vi "9239_1 - test.vi"() -> ()   [LabVIEW 2014]
uses:
  <vilib>/Platform/TimedLoop/XDataNode/timing_clust.ctl
  <vilib>/Platform/TimedLoop/XDataNode/nitl_modes.ctl
  <vilib>/Platform/TimedLoop/XDataNode/wakeup.ctl
  <vilib>/Platform/TimedLoop/XDataNode/XDataNode.xnode
  <vilib>/Platform/TimedLoop/XDataNode/XDNodeRunTimeDep.lvlib
panel:
  out "已采样数量":dbl
  out "a1通道零漂采集":dynamicdata(graph)
  in  "路径":path=path "test"
  out "波形图":dynamicdata(graph)
  out "时间":string
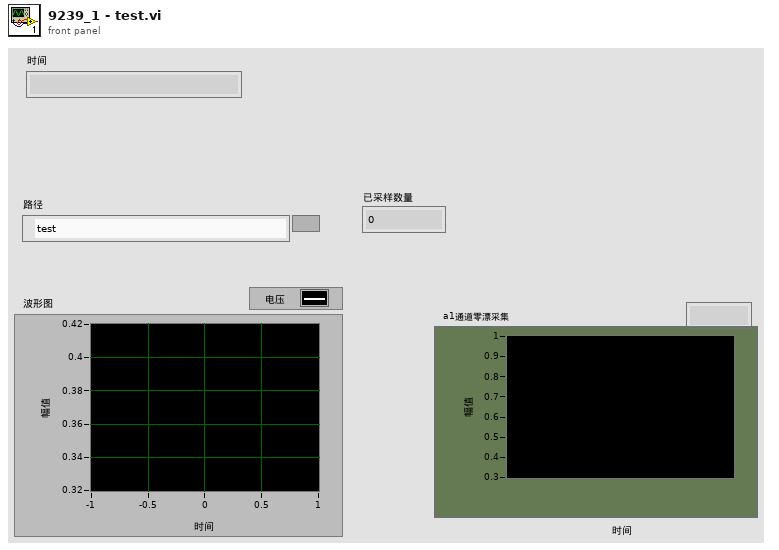
[diagram p1: front panel]
types:
  T1 = enum16{"open", "open or create", "create or replace", "create", "open (read-only)"}
  T2 = typedef "XDNodeRunTimeDep.lvlib/timing_clust.ctl" = cluster{"Expected End [f-1]":u64, "Actual End [f-1]":u64, "Finished Late? [f-1]":bool, "Expected End [i-1]":u64, "Actual End [i-1]":u64, "Finished Late? [i-1]":bool, "Expected Start [i]":u64, "Actual Start [i]":u64, "Expected Start [f]":u64, "Actual Start [f]":u64, "Source Name":string, "Structure Name":string, "Period":i64, "Deadline":i64, "Offset":i64, "Start":i64, "Priority":i32, "Timeout":i32, "Mode":T3, "Wakeup Reason":T4, "Error":errorcluster, "Source Type":string, "Secondary Source Type":string, "Global End Time":u64, "Global Start Time":u64, "Frame Duration":u64, "Iteration Duration":u64, "Assigned CPU":i32, "I/O Scan Engine Mode":u32}
  T3 = typedef "XDNodeRunTimeDep.lvlib/nitl_modes.ctl" = enum32{"No Change", "Process missed periods, maintain original phase", "Discard missed periods, maintain original phase", "Process missed periods, ignore original phase", "Discard missed periods, ignore original phase"}
  T4 = typedef "XDNodeRunTimeDep.lvlib/wakeup.ctl" = enum32{"Normal", "Aborted", "Asynchronous wakeup", "Timing source error", "Timed loop error", "Timeout"}
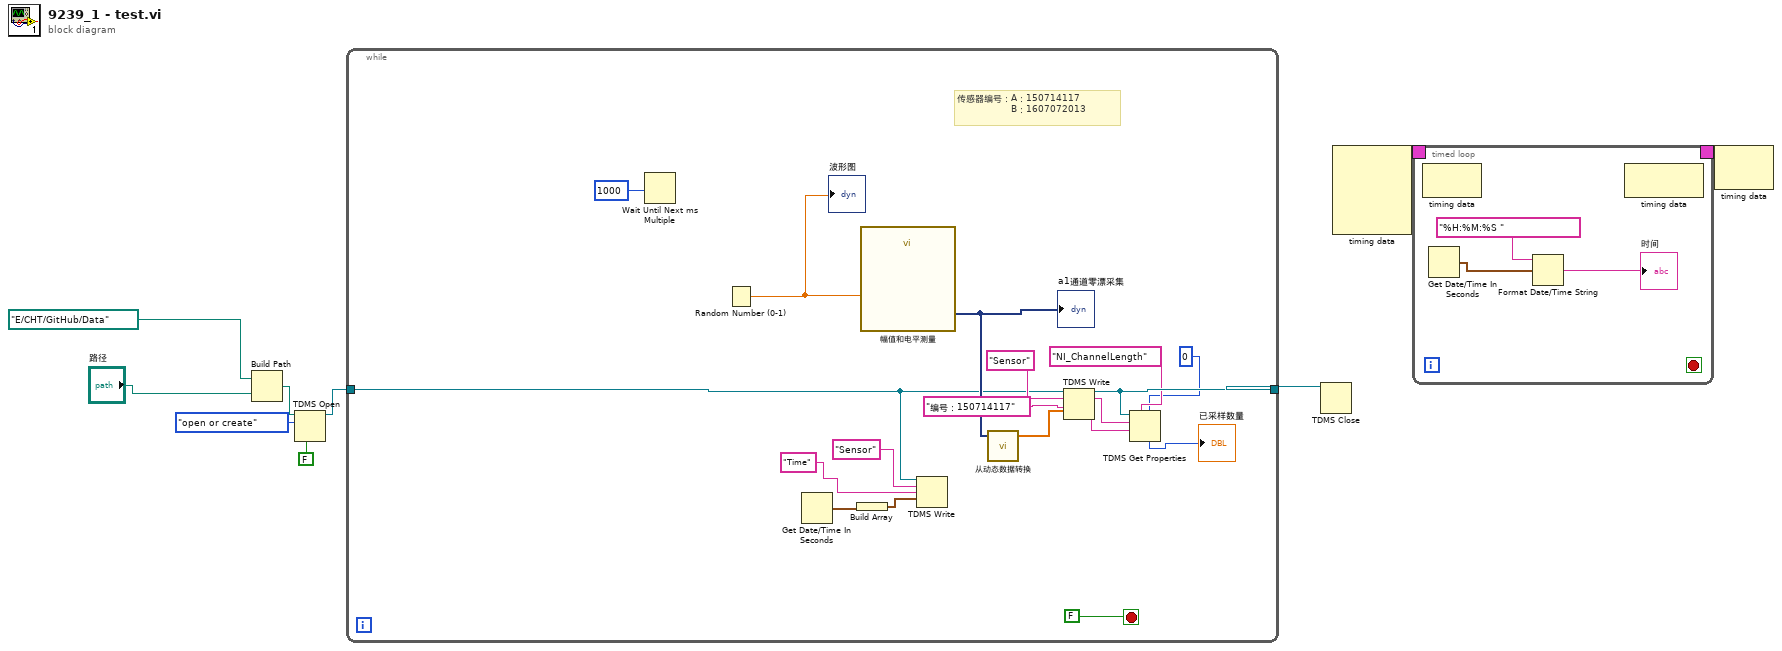
[diagram p0: block diagram]
diagram:
  n1 = Build Path(base path=path "E:/CHT/GitHub/Data", name or relative path="路径") -> (appended path=w6:path)
  n2 = TDMS Open(6:FALSE ("disable buffering (T)"), 10:T1."open or create" ("operation"), 11:w6) -> (3:w4:refnum<k34>)  [unwired: 4 in, 1 out]
  n3 = while {
    tunnel: w4 -> [w14]
    tunnel: [w21] -> w3
    stop <- FALSE stop-if-true
    # "传感器编号：A：150714117\n                  B：1607072013"
    n4 = Wait Until Next ms Multiple(millisecond multiple=1000) -> ()  [unwired: 1 out]
    n5 = Random Number (0-1)() -> (number: 0 to 1=w11:dbl)
    "波形图" <- w11
    n6 = Get Date/Time In Seconds() -> (seconds since 1Jan1904=w16:timestamp)
    n7 = Build Array(w16) -> (w15:timestamp[])
    n8 = call "幅值和电平测量"("Signals"=w11) -> ("Mean (DC)"=w24:dynamicdata)  [unwired: 13 in, 1 out]
    "a1通道零漂采集" <- w24
    n9 = TDMS Write(0:w14, 5:"Sensor", 7:"Time", 9:w15) -> ()  [unwired: 2 in, 4 out]
    n10 = call "从动态数据转换"("Dynamic Data Type"=w24) -> ("Array"=w23:dbl[])  [unwired: 3 in]
    n11 = TDMS Write(0:w14, 5:"Sensor", 7:"编号：150714117", 9:w23) -> (4:w21:refnum<k34>, 6:w22:string, 8:w20:string)  [unwired: 2 in, 1 out]
    n12 = TDMS Get Properties(5:0, 7:"NI_ChannelLength", 9:w20, 10:w22, 11:w21) -> (4:→"已采样数量":i32)  [unwired: 1 in, 5 out]
  }
  n13 = TDMS Close(11:w3) -> ()  [unwired: 1 in, 2 out]
  n14 = node-c288() -> (w9:T2)  [unwired: 4 in]
  n15 = timed-loop {
    timing: w9 -> [_]
    timing-out: [_] -> w8
    stop <- _ stop-if-true
    n16 = node-c288() -> ()  [unwired: 1 in, 1 out]
    n17 = Get Date/Time In Seconds() -> (seconds since 1Jan1904=w30:timestamp)
    n18 = Format Date/Time String(time format string (%c)="%H:%M:%S ", seconds (now)=w30) -> (date/time string=→"时间":string)  [unwired: 1 in]
    n19 = node-c288() -> ()  [unwired: 1 in, 1 out]
  }
  n20 = node-c288(w8) -> ()  [unwired: 1 out]
